vi "单位换算.vi"() -> ()   [LabVIEW 2013]
panel:
  in  "确定按钮":bool
  in  "单位 4":u16(ring) items=["周", "天", "年", "微妙", "毫秒", "秒", "分", "小时"]
  in  "单位":u16(ring) items=["周", "天", "年", "微妙", "毫秒", "秒", "分", "小时"]
  in  "数值 6":dbl
  in  "数值 5":dbl
  in  "单位 3":u16(ring) items=["分", "钱", "两", "斤", "担", "吨", "微克", "毫克", "克拉", "克", "千克"]
  in  "数值 4":dbl
  in  "单位":u16(ring) items=["分", "钱", "两", "斤", "担", "吨", "微克", "毫克", "克拉", "克", "千克"]
  in  "数值 3":dbl
  in  "单位 2":u16(ring) items=["毫", "里", "分", "寸", "尺", "丈", "里", "分米", "厘米", "千米", "皮米", "纳米", "微米", "毫米", "米", ""]
  in  "数值 2":dbl
  in  "数值":dbl
  in  "单位":u16(ring) items=["毫", "里", "分", "寸", "尺", "丈", "里", "分米", "厘米", "千米", "皮米", "纳米", "微米", "毫米", "米"]
  # "长度"
  # "质量"
  # "时间"
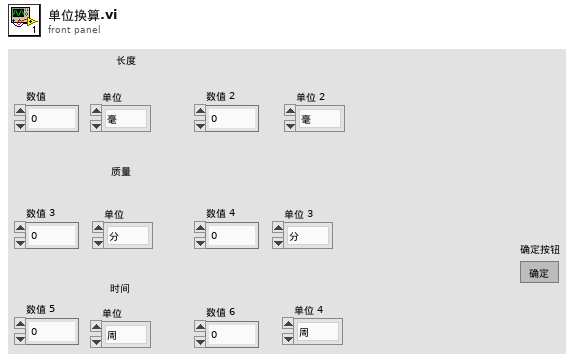
[diagram p1: front panel]
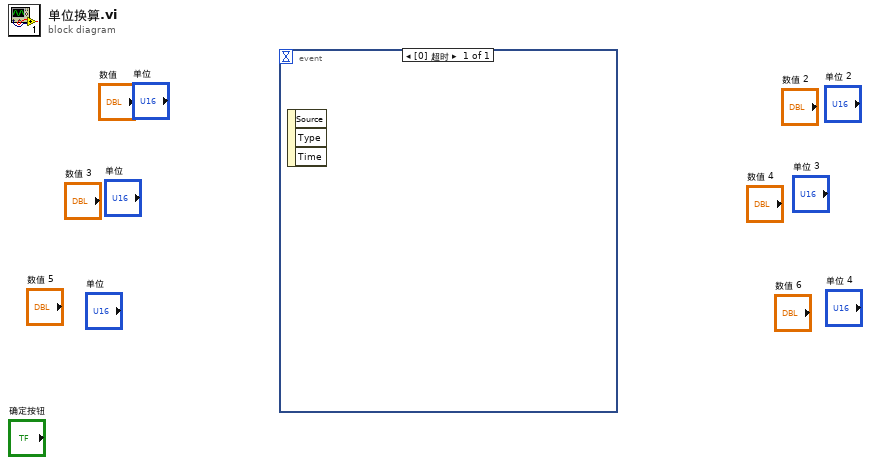
[diagram p0: block diagram]
diagram:
  n1 = event shown="[0] 超时" {
    selector: _ -> [_]
    dyn-events: _ -> [_]
    timeout: _ -> [_]
    event Timeout {
      n2 = event-data() -> ()  [unwired: 1 in, 3 out]
    }
  }
